vi "GetRandomNum.vi"(8 "error in (no error)":errorcluster, 11 "Generator in":refnum<class "Generator.lvclass">) -> (0 "error out":errorcluster, 3 "Generator out":refnum<class "Generator.lvclass">)   [LabVIEW 2021, in "Generator.lvlib" / "Generator.lvclass"]
uses:
  Generator.lvclass
  Generator.lvclass/Generator.ctl
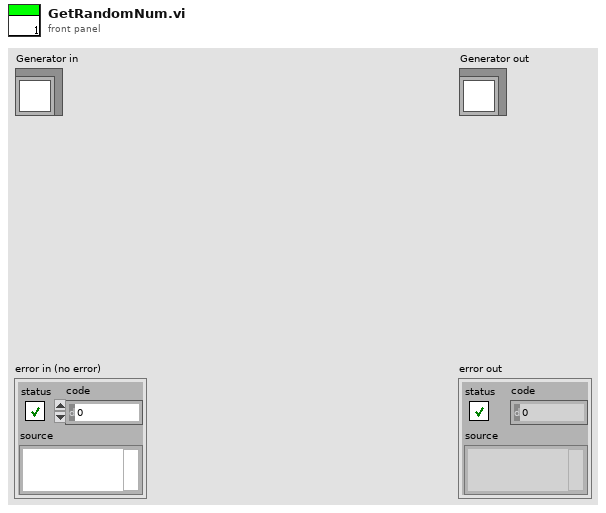
[diagram p1: front panel]
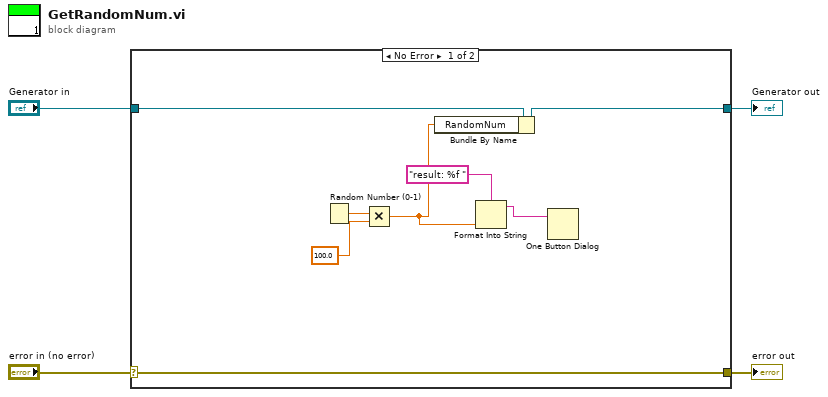
[diagram p0: block diagram]
diagram:
  n1 = case shown="No Error" "error in (no error)" {
    selector: "error in (no error)" -> [w11 w14]
    tunnel: [w11 w14] -> w3
    tunnel: [w8 w13] -> w1
    tunnel: "Generator in" -> [w12 w13]
    frame No Error {
      n2 = Random Number (0-1)() -> (number: 0 to 1=w10:dbl)
      n3 = Multiply(x=w10, y=100.0) -> (x*y=w5:dbl)
      n4 = Bundle By Name(cluster=w12, "RandomNum"=w5) -> (w8:refnum<class "Generator.lvclass">)
      n5 = Format Into String(format string="result: %f ", w5) -> (resulting string=w7:string)  [unwired: 2 in, 1 out]
      n6 = One Button Dialog(message=w7) -> ()  [unwired: 1 in, 1 out]
    }
    frame Error {
    }
  }
  "error out" <- w3
  "Generator out" <- w1
